vi "Shooter Controller.vi"(8 "error in":errorcluster) -> ()   [LabVIEW 2025]
doc: "This VI executes continuously carrying out the current operation and responding to updates or new operations. It will often contain the timing or control code that is difficult to place directly in TeleOp. This VI generally opens all sensors and motors and isolates the rest of the robot code from knowing how the operations are carried out."
uses:
  <vilib>/Rock Robotics/WPI/Framework/Completion Status.ctl
  Shooter Setpoints.ctl
  Shooter Operations.ctl
  swerve-template/Type Definitions/Data/Robot Velocities.ctl
  <vilib>/Rock Robotics/WPI/ThirdParty/REV Robotics/REVLib/Typedef/SPARK PID Gains.ctl
  <vilib>/Rock Robotics/WPI/ThirdParty/REV Robotics/REVLib/Typedef/SPARK Feed Forward Gains.ctl
  <vilib>/Rock Robotics/WPI/ThirdParty/REV Robotics/REVLib/Typedef/Spark MAX Idle Mode.ctl
  <vilib>/Rock Robotics/WPI/ThirdParty/REV Robotics/REVLib/Typedef/Spark MAX Control Type.ctl
  a69457f0-b09a-4d5a-aa11-90b3f8aeabef.vi
  369ad276-722f-42d5-b4e5-f74530a454e4.vi
  <vilib>/Rock Robotics/WPI/ThirdParty/REV Robotics/REVLib/SubVI/Public/SPARK Open Brushless.vi
  <vilib>/Rock Robotics/WPI/ThirdParty/REV Robotics/REVLib/SubVI/Public/SPARK Configure Soft Limit Reverse.vi
  <vilib>/Rock Robotics/WPI/ThirdParty/REV Robotics/REVLib/SubVI/Public/SPARK Configure Soft Limit Forward.vi
  <vilib>/Rock Robotics/WPI/ThirdParty/REV Robotics/REVLib/SubVI/Public/SPARK Configure Closed Loop Gains.vi
  <vilib>/Rock Robotics/WPI/ThirdParty/REV Robotics/REVLib/SubVI/Public/SPARK Configure Basic Idle Mode.vi
  <vilib>/Rock Robotics/WPI/ThirdParty/REV Robotics/REVLib/SubVI/Public/SPARK Configure Power Current Limit.vi
  <vilib>/Rock Robotics/WPI/ThirdParty/REV Robotics/REVLib/SubVI/Public/SPARK Get Encoder Status Position.vi
  <vilib>/Rock Robotics/Network Tables/NT Read Float Array.vi
  <vilib>/Rock Robotics/WPI/ThirdParty/REV Robotics/REVLib/SubVI/Public/SPARK Configure Follower Mode From Ref.vi
  <vilib>/Rock Robotics/Network Tables/NT Write Boolean.vi
panel:
  out "Shooter Hood":dbl(graph)
  in  "Hood FF":T1
  in  "Hood PID":T2
  in  "Shooter FF":T1={"kV"=0.00185, "kS"=0.0, "kA"=0.0, "kG"=0.0, "kCos"=0.0, "kCosRatio"=0.0}
  in  "Shooter PID":T2
  in  "Interactive Values":T3
  out "Current\nCmd":string
  in  "Buttons":cluster{"Execute Cmd":bool, "Abort Cmd":bool}
  out "Command Timing":cluster{"Start Time (ms)":u32, "Iterations":i32}
  out "Status":T6
  # "Interactive Command: You may fill in the settings for a command\nand schedule it with the Execute button. You can observe and abort\nany command while fine tuning the code for the controller."
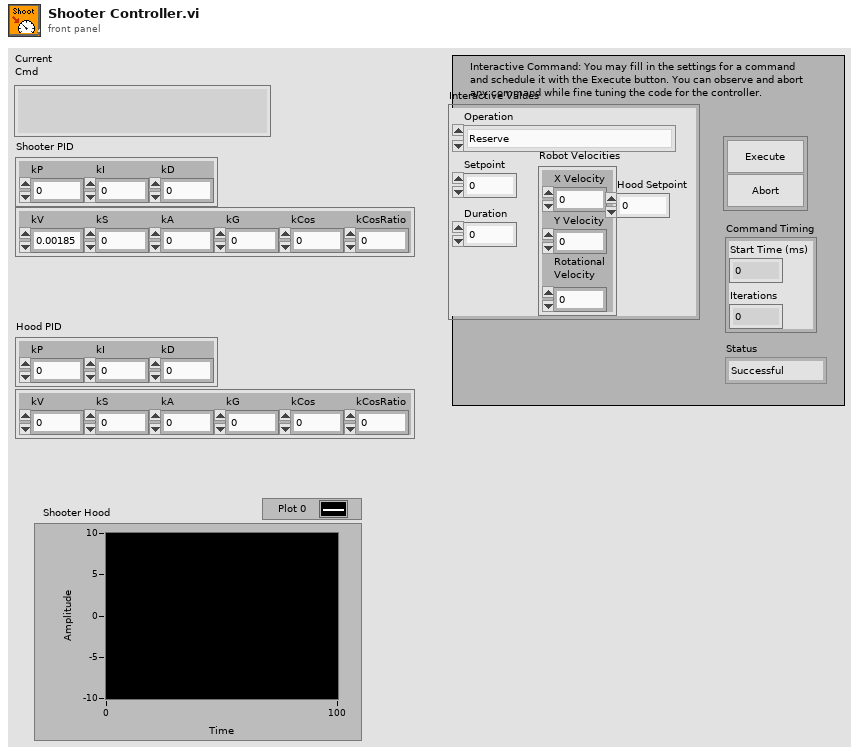
[diagram p1: front panel]
types:
  T1 = typedef "SPARK Feed Forward Gains.ctl" = cluster{"kV":dbl, "kS":dbl, "kA":dbl, "kG":dbl, "kCos":dbl, "kCosRatio":dbl}
  T2 = typedef "SPARK PID Gains.ctl" = cluster{"kP":dbl, "kI":dbl, "kD":dbl}
  T3 = typedef "Shooter Setpoints.ctl" = cluster{"Operation":T4, "Setpoint":dbl, "Duration":dbl, "Robot Velocities":T5, "Hood Setpoint":dbl}
  T4 = typedef "Shooter Operations.ctl" = enum16{"Reserve", "Read Current", "Interpolated Shot", "Hood Manual", "Reset Hood", "Immediate"}
  T5 = typedef "Robot Velocities.ctl" = cluster{"X Velocity":dbl, "Y Velocity":dbl, "Rotational \nVelocity":dbl}
  T6 = typedef "Completion Status.ctl" = enum16{"Successful", "Aborted", "Incomplete"}
  T7 = typedef "Spark MAX Idle Mode.ctl" = enum16{"Coast", "Brake"}
  T8 = typedef "WPI_MotorControlDeviceRef.ctl" = cluster{"DeviceStatus":errorcluster, "Type":T9, "PWM":cluster{"PWM Channel":T10, "DeadBand":T11}, "CAN":cluster{"Device Number":u8, "SetOutput VI Ref":variant, "GetOutput VI Ref":variant, "Enable VI Ref":variant, "Disable VI Ref":variant, "Data":variant}, "Invert":bool, "DIO PWM":cluster{"PWM \"Enable\" Channel":T10, "DIOChannel":T12, "PWM Rate":dbl}}
  T9 = typedef "WPI_MotorControlType.ctl" = enum16{"PWM", "CAN", "DIO PWM"}
  T10 = typedef "FPGA_DIOPWMChannel.ctl" = enum8{"PWM 0", "PWM 1", "PWM 2", "PWM 3", "PWM 4", "PWM 5", "PWM 6", "PWM 7", "PWM 8", "PWM 9", "PWM MXP 0", "PWM MXP 1", "PWM MXP 2", "PWM MXP 3", "PWM MXP 4", "PWM MXP 5", "PWM MXP 6", "PWM MXP 7", "PWM MXP 8", "PWM MXP 9", "Invalid"}
  T11 = typedef "WPI_PWMDeadband.ctl" = cluster{"Name":string, "maxPositivePwm":i32, "minPositivePwm":i32, "centerPwm":i32, "maxNegativePwm":i32, "minNegativePwm":i32, "angularRange":u16}
  T12 = typedef "FPGA_DIOChannel.ctl" = enum8{"DIO 0", "DIO 1", "DIO 2", "DIO 3", "DIO 4", "DIO 5", "DIO 6", "DIO 7", "DIO 8", "DIO 9", "DIO MXP 0", "DIO MXP 1", "DIO MXP 2", "DIO MXP 3", "DIO MXP 4", "DIO MXP 5", "DIO MXP 6", "DIO MXP 7", "DIO MXP 8", "DIO MXP 9", "DIO MXP 10", "DIO MXP 11", "DIO MXP 12", "DIO MXP 13", "DIO MXP 14", "DIO MXP 15", "SPI Port CS1", "SPI Port CS2", "SPI Port CS3", "SPI Port MISO", "SPI Port MOSI", "Invalid"}
  T13 = typedef "Command Status Info.ctl" = cluster{"Name":string, "Status":T6, "notifier out":T14}
  T14 = typedef "Completion Notifier.ctl" = refnum<notifier>
  T15 = cluster{"Current Command":T3, "Command Timing":cluster{"Start Time (ms)":u32, "Iterations":i32}, "Command Arguments":cluster{"Command Info":T13, "Description":string, "Default Command":T3, "queue out":refnum<queue>, "Subsystem Name":string}}
  T16 = typedef "Spark MAX Control Type.ctl" = enum16{"Percent VBus", "Voltage", "Velocity", "Position", "Smart Motion", "Current", "Smart Velocity", "MAXMotion Position", "MAXMotion Velocity"}
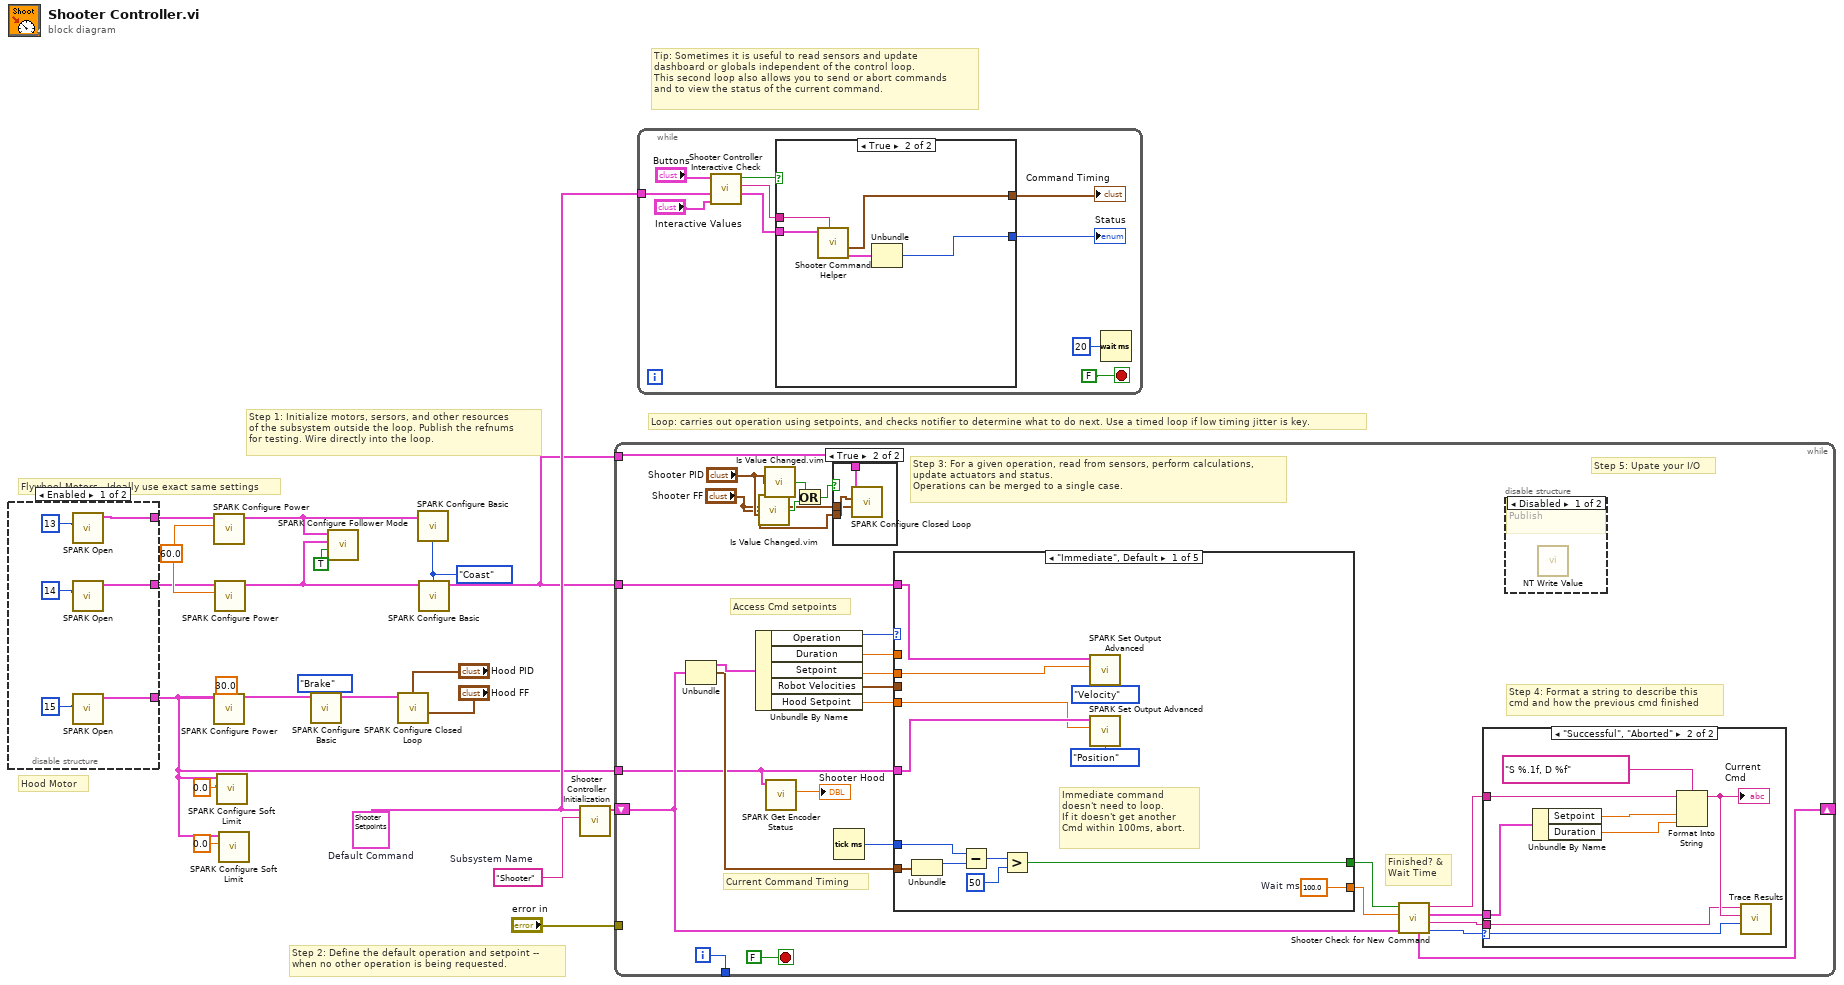
[diagram p0: block diagram]
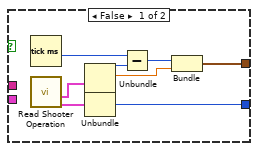
[diagram p3: hidden frame]
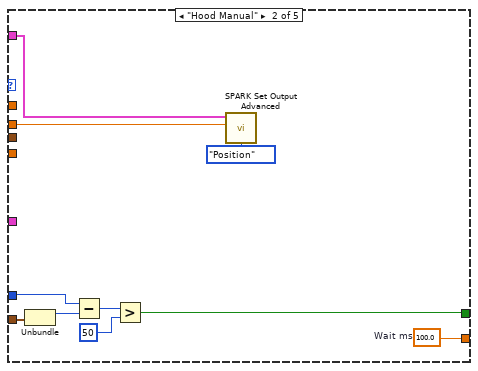
[diagram p7: hidden frame]
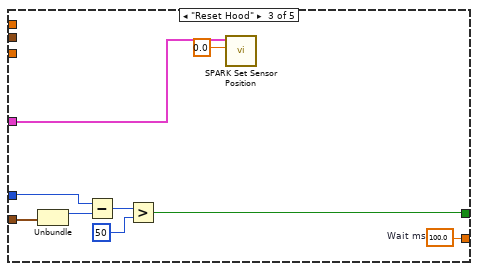
[diagram p8: hidden frame]
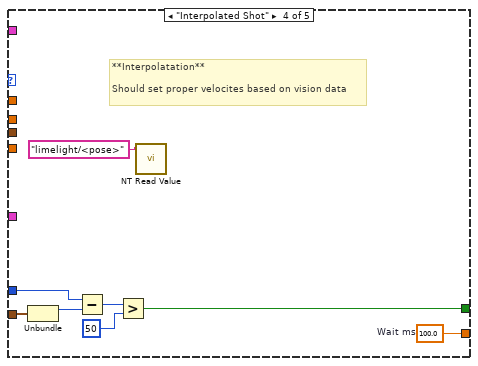
[diagram p9: hidden frame]
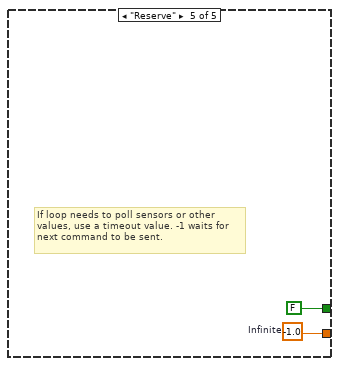
[diagram p10: hidden frame]
diagram:
  w10 = Spark_MAX_Idle_Mode."Coast" ("Idle Mode")
  w12 = sgl 60.0 ("Current Limit A (100)")
  w13 = T3 {"Operation"=enum."Reserve", "Setpoint"=0.0, "Duration"=0.0, "Robot Velocities"={"X Velocity"=0.0, "Y Velocity"=0.0, "Rotational \nVelocity"=0.0}, "Hood Setpoint"=0.0}  # Default Command
  w14 = "Shooter"  # Subsystem Name
  # "Hood Motor"
  # "Flywheel Motors - Ideally use exact same settings"
  # "Tip: Sometimes it is useful to read sensors and update\ndashboard or globals independent of the control loop.\nThis second loop also allows you to send or abort commands\nand to view the status of the current command."
  # "Step 2: Define the default operation and setpoint --\nwhen no other operation is being requested."
  # "Step 1: Initialize motors, sersors, and other resources\nof the subsystem outside the loop. Publish the refnums\nfor testing. Wire directly into the loop."
  # "Loop: carries out operation using setpoints, and checks notifier to determine what to do next. Use a timed loop if low timing jitter is key."
  n1 = disable-structure shown="Enabled" {
    disable-tunnel: [w19 _] -> w7
    disable-tunnel: [w18 _] -> w11
    disable-tunnel: [w17 _] -> w1
    frame Enabled {
      n2 = call-poly <vilib>:"SPARK Open.vi"("Device Number"=u8 13) -> ("MotorControlDeviceRef"=w18:T8)  [unwired: 9 in, 1 out]
      n3 = call-poly <vilib>:"SPARK Open.vi"("Device Number"=u8 14) -> ("MotorControlDeviceRef"=w19:T8)  [unwired: 9 in, 1 out]
      n4 = call-poly <vilib>:"SPARK Open.vi"("Device Number"=u8 15) -> ("MotorControlDeviceRef"=w17:T8)  [unwired: 9 in, 1 out]
    }
    frame Disabled {
    }
  }
  n5 = call-poly <vilib>:"SPARK Configure Power.vi"("Current Limit A (100)"=w12, "MotorControlDeviceRef in"=w11) -> ()  [unwired: 8 in, 2 out]
  n6 = call-poly <vilib>:"SPARK Configure Power.vi"("Current Limit A (100)"=sgl 30.0, "MotorControlDeviceRef in"=w1) -> ()  [unwired: 8 in, 2 out]
  n7 = call-poly <vilib>:"SPARK Configure Power.vi"("Current Limit A (100)"=w12, "MotorControlDeviceRef in"=w7) -> ()  [unwired: 8 in, 2 out]
  n8 = call-poly <vilib>:"SPARK Configure Soft Limit.vi"("Soft Limit"=0.0, "MotorControlDeviceRef in"=w1) -> ()  [unwired: 8 in, 2 out]
  n9 = call-poly <vilib>:"SPARK Configure Soft Limit.vi"("Soft Limit"=0.0, "MotorControlDeviceRef in"=w1) -> ()  [unwired: 8 in, 2 out]
  n10 = call-poly <vilib>:"SPARK Configure Basic.vi"("Idle Mode"=Spark_MAX_Idle_Mode."Brake", "MotorControlDeviceRef in"=w1) -> ()  [unwired: 8 in, 2 out]
  n11 = call-poly <vilib>:"SPARK Configure Follower Mode.vi"("Invert From Leader"=TRUE, "Leader MotorControlDeviceRef"=w7, "MotorControlDeviceRef in"=w11) -> ()  [unwired: 7 in, 2 out]
  n12 = call-poly <vilib>:"SPARK Configure Closed Loop.vi"("Feed Forward Gains"="Hood FF", "PID Gains"="Hood PID", "MotorControlDeviceRef in"=w1) -> ()  [unwired: 7 in, 2 out]
  n13 = call-poly <vilib>:"SPARK Configure Basic.vi"("Idle Mode"=w10, "MotorControlDeviceRef in"=w11) -> ()  [unwired: 8 in, 2 out]
  n14 = call-poly <vilib>:"SPARK Configure Basic.vi"("Idle Mode"=w10, "MotorControlDeviceRef in"=w7) -> ()  [unwired: 8 in, 2 out]
  n15 = call "Shooter Controller Initialization.vi"("Subsystem Name"=w14, "Default Command"=w13) -> ("Current Command"=w15:T15)  [unwired: 9 in]
  n16 = while {
    shift-right: [w41] -> _
    shift-left: w15 -> [w34]
    tunnel: [w48] -> _
    tunnel: "error in" -> [_]
    tunnel: w7 -> [w27]
    tunnel: w7 -> [w26]
    tunnel: w1 -> [w24]
    i -> [w48]
    stop <- FALSE stop-if-true
    # "Step 5: Upate your I/O"
    # "Step 4: Format a string to describe this\ncmd and how the previous cmd finished"
    # "Current Command Timing"
    # "Access Cmd setpoints"
    # "Finished? &\nWait Time"
    # "Step 3: For a given operation, read from sensors, perform calculations,\nupdate actuators and status.\nOperations can be merged to a single case."
    n17 = Unbundle(w34) -> ("Current Command"=w47:T3, "Command Timing"=w43:cluster{"Start Time (ms)":u32, "Iterations":i32})  [unwired: 1 out]
    n18 = Unbundle By Name(w47) -> ("Operation"=w46:T4, "Duration"=w45:dbl, "Setpoint"=w42:dbl, "Robot Velocities"=w33:T5, "Hood Setpoint"=w25:dbl)
    n19 = call "Is Value Changed.vim"("value"="Shooter FF") -> ("changed or first call?"=w31:bool)
    n20 = call "Is Value Changed.vim"("value"="Shooter PID") -> ("changed or first call?"=w32:bool)
    n21 = call-poly <vilib>:"SPARK Get Encoder Status.vi"("MotorControlDevRef in"=w24) -> ("Sensor Position"=→"Shooter Hood":dbl)  [unwired: 7 in, 3 out]
    n22 = Or(x=w32, y=w31) -> (x .or. y?=w30:bool)
    n23 = case shown="True" w30 {
      tunnel: w27 -> [_ w52]
      tunnel: "Shooter PID" -> [_ w51]
      tunnel: "Shooter FF" -> [_ w50]
      frame False {
      }
      frame True {
        n24 = call-poly <vilib>:"SPARK Configure Closed Loop.vi"("Feed Forward Gains"=w50, "PID Gains"=w51, "MotorControlDeviceRef in"=w52) -> ()  [unwired: 7 in, 2 out]
      }
    }
    n25 = Tick Count (ms)() -> (millisecond timer value=w44:u32)
    n26 = case shown="\"Immediate\", Default" w46 {
      tunnel: [w73 w74 w84 w94 w102] -> w39
      tunnel: [w67 w75 w85 w95 FALSE ("ignore previous (F)")] -> w40
      tunnel: w43 -> [w69 w76 w86 w97 _]
      tunnel: w45 -> [_ _ _ _ _]
      tunnel: w44 -> [w68 w77 w87 w96 _]
      tunnel: w42 -> [w64 w82 _ _ _]
      tunnel: w33 -> [_ _ _ _ _]
      tunnel: w26 -> [w65 w81 _ _ _]
      tunnel: w25 -> [w61 _ _ _ _]
      tunnel: w24 -> [w62 _ w92 _ _]
      frame "Immediate", Default {
        w73 = 100.0  # Wait ms
        # "Immediate command\ndoesn't need to loop.\nIf it doesn't get another\nCmd within 100ms, abort."
        n27 = Unbundle(w69) -> ("Start Time (ms)"=w72:u32)  [unwired: 1 out]
        n28 = Subtract(x=w68, y=w72) -> (x-y=w71:u32)
        n29 = Greater?(x=w71, y=u8 50 ("Left Motor")) -> (0:w67:bool)
        n30 = call <vilib>:"SPARK Set Output Advanced.vi"("Control Mode"=Spark_MAX_Control_Type."Velocity", "Setpoint"=w64, "MotorControlDevRef"=w65) -> ()  [unwired: 7 in, 2 out]
        n31 = call <vilib>:"SPARK Set Output Advanced.vi"("Control Mode"=Spark_MAX_Control_Type."Position", "Setpoint"=w61, "MotorControlDevRef"=w62) -> ()  [unwired: 7 in, 2 out]
      }
      frame "Hood Manual" {
        w74 = 100.0  # Wait ms
        n32 = Unbundle(w76) -> ("Start Time (ms)"=w80:u32)  [unwired: 1 out]
        n33 = Subtract(x=w77, y=w80) -> (x-y=w79:u32)
        n34 = Greater?(x=w79, y=u8 50 ("Left Motor")) -> (0:w75:bool)
        n35 = call <vilib>:"SPARK Set Output Advanced.vi"("Control Mode"=Spark_MAX_Control_Type."Position", "Setpoint"=w82, "MotorControlDevRef"=w81) -> ()  [unwired: 7 in, 2 out]
      }
      frame "Reset Hood" {
        w84 = 100.0  # Wait ms
        n36 = Unbundle(w86) -> ("Start Time (ms)"=w90:u32)  [unwired: 1 out]
        n37 = Subtract(x=w87, y=w90) -> (x-y=w89:u32)
        n38 = Greater?(x=w89, y=u8 50 ("Left Motor")) -> (0:w85:bool)
        n39 = call <vilib>:"SPARK Set Sensor Position.vi"("Position"=0.0, "MotorControlDeviceRef"=w92) -> ()  [unwired: 8 in, 2 out]
      }
      frame "Interpolated Shot" {
        w94 = 100.0  # Wait ms
        # "**Interpolatation**\n\nShould set proper velocites based on vision data"
        n40 = Unbundle(w97) -> ("Start Time (ms)"=w100:u32)  [unwired: 1 out]
        n41 = Subtract(x=w96, y=w100) -> (x-y=w99:u32)
        n42 = Greater?(x=w99, y=u8 50 ("Left Motor")) -> (0:w95:bool)
        n43 = call-poly <vilib>:"NT Read Value.vi"("name"="limelight/<pose>") -> ()  [unwired: 8 in, 3 out]
      }
      frame "Reserve" {
        w102 = -1.0  # Infinite
        # "If loop needs to poll sensors or other\nvalues, use a timeout value. -1 waits for\nnext command to be sent."
      }
    }
    n44 = call "Shooter Check for New Command.vi"("Current Command"=w34, "Wait time (ms)"=w39, "Finished?"=w40) -> ("Completion"=w35:T6, "Subsystem Name"=w36:string, "Current Command"=w37:T3, "Initial Trace String"=w38:string, "NextCommand"=w41:T15)  [unwired: 4 in]
    n45 = case shown="\"Successful\", \"Aborted\"" w35 {
      selector: w35 -> [_ w60]
      tunnel: w38 -> [_ w56]
      tunnel: w37 -> [_ w57]
      tunnel: w36 -> [_ w53]
      frame "Incomplete", Default {
        # "Continuing current command"
      }
      frame "Successful", "Aborted" {
        # "Report and setup for next command"
        n46 = Unbundle By Name(w57) -> ("Setpoint"=w59:dbl, "Duration"=w54:dbl)
        n47 = Format Into String(format string="S %.1f, D %f", initial string=w56, w59, w54) -> (resulting string=w55:string)  [unwired: 1 in, 1 out]
        "Current\nCmd" <- w55
        n48 = call <vilib>:"Trace Results.vi"("Status of previous command"=w60, "Description"=w55, "Subsystem"=w53) -> ()  [unwired: 9 in]
      }
    }
    n49 = disable-structure shown="Disabled" {
      frame Disabled {
        # "Publish"
        n50 = call-poly <vilib>:"NT Write Value.vi"() -> ()  [unwired: 11 in, 1 out]
      }
      frame Enabled {
      }
    }
  }
  n51 = while {
    tunnel: w13 -> [w109]
    stop <- FALSE stop-if-true
    n52 = call "Shooter Controller Interactive Check.vi"("Interactive Command in"="Interactive Values", "Default Command"=w109, "Buttons"="Buttons") -> ("Interactive Command out"=w106:T3, "Trace String"=w107:string, "Schedule"=w108:bool)  [unwired: 6 in]
    n53 = case shown="True" w108 {
      tunnel: [w120 w125] -> w105
      tunnel: w106 -> [_ w123]
      tunnel: [w116 w121] -> w104
      tunnel: w107 -> [_ w124]
      frame False {
        n54 = Tick Count (ms)() -> (millisecond timer value=w115:u32)
        n55 = call "Read Shooter Operation.vi"() -> ("Command Info"=w113:T13, "SubSystem Data"=w114:T3)  [unwired: 9 in, 1 out]
        n56 = Unbundle(w114) -> ("Operation"=w119:T4, "Setpoint"=w117:dbl)  [unwired: 3 out]
        n57 = Unbundle(w113) -> ("Status"=w120:T6)  [unwired: 2 out]
        n58 = Subtract(x=w115, y=w119) -> (x-y=w118:u32)
        n59 = Bundle(w118, "Setpoint"=w117) -> (w116:cluster{u32, "Setpoint":dbl})  [unwired: 1 in]
      }
      frame True {
        n60 = call "Shooter Command Helper.vi"("Description"=w124, "SubSystem Data"=w123) -> ("Command Info Out"=w122:T13, "Command Timing"=w121:cluster{"Start Time (ms)":u32, "Iterations":i32})  [unwired: 7 in, 1 out]
        n61 = Unbundle(w122) -> ("Status"=w125:T6)  [unwired: 2 out]
      }
    }
    "Status" <- w105
    "Command Timing" <- w104
    n62 = Wait (ms)(milliseconds to wait=u32 20) -> ()  [unwired: 1 out]
  }
